vi "is_experiment_finished.vi"(8 "error in (no error)":errorcluster, 11 "DL090430TriggeredExperimentController.lvclass in":refnum<class "ExperimentControllerDL090803Triggered.lvclass">) -> (0 "error out":errorcluster, 2 "experiment finished?":bool, 3 "DL090430TriggeredExperimentController.lvclass out":refnum<class "ExperimentControllerDL090803Triggered.lvclass">)   [LabVIEW 2010, in "ExperimentControllerDL090803Triggered.lvclass"]
uses:
  ExperimentControllerDL090803Triggered.lvclass
  ExperimentControllerDL090803Triggered.lvclass/ExperimentControllerDL090803Triggered.ctl
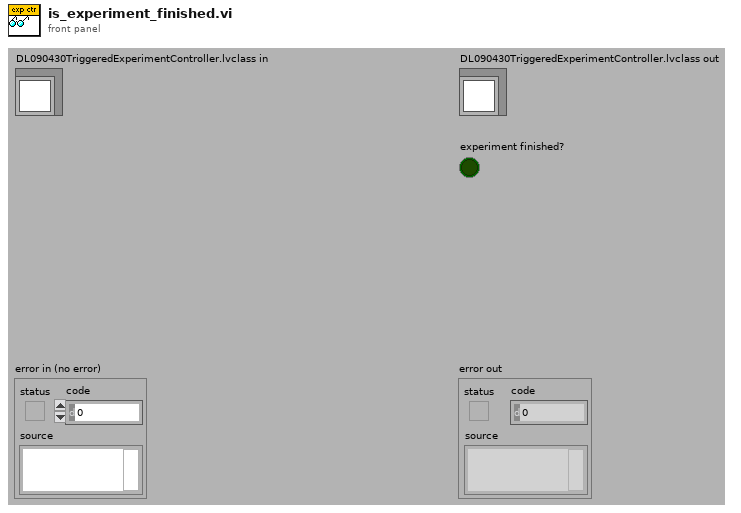
[diagram p1: front panel]
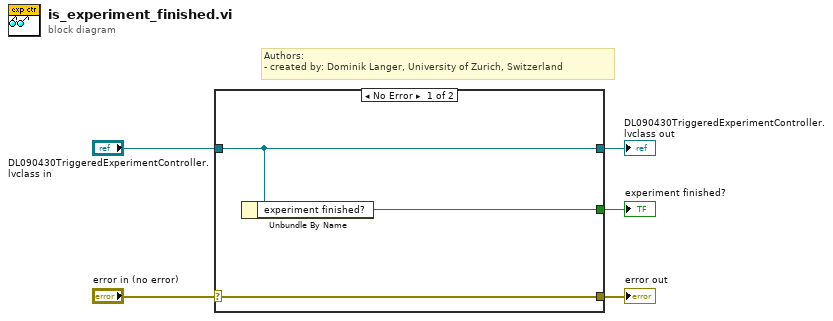
[diagram p0: block diagram]
diagram:
  # "Authors: \n- created by: Dominik Langer, University of Zurich, Switzerland"
  n1 = case shown="No Error" "error in (no error)" {
    selector: "error in (no error)" -> [w8 w9]
    tunnel: [w8 w9] -> w4
    tunnel: [w7 w10] -> w2
    tunnel: "DL090430TriggeredExperimentController.lvclass in" -> [w7 w10]
    tunnel: [w6 _] -> w1
    frame No Error {
      n2 = Unbundle By Name(w7) -> ("experiment finished?"=w6:bool)
    }
    frame Error {
    }
  }
  "error out" <- w4
  "DL090430TriggeredExperimentController.lvclass out" <- w2
  "experiment finished?" <- w1
